vi "Stiffness Limits DAO.vi"(0 "Actions":T5, 3 "Config Ref Number":T4, 7 "ID":T3, 9 "Stiffness Limit In":T1, 11 "error in (no error)":errorcluster) -> (8 "Stiffness Limit Out":T1, 14 "Config Ref Number out":T4, 15 "error out":errorcluster)   [LabVIEW 2013]
uses:
  Metadata/Persistant DAO Actions.ctl
  <vilib>/Utility/config.llb/Config Data RefNum.ctl
  Metadata/LBCB Number.ctl
  Metadata/Cartesian Matrix.ctl
  Metadata/Cartesian Point.ctl
  <vilib>/Utility/config.llb/NI_LVConfig.lvlib
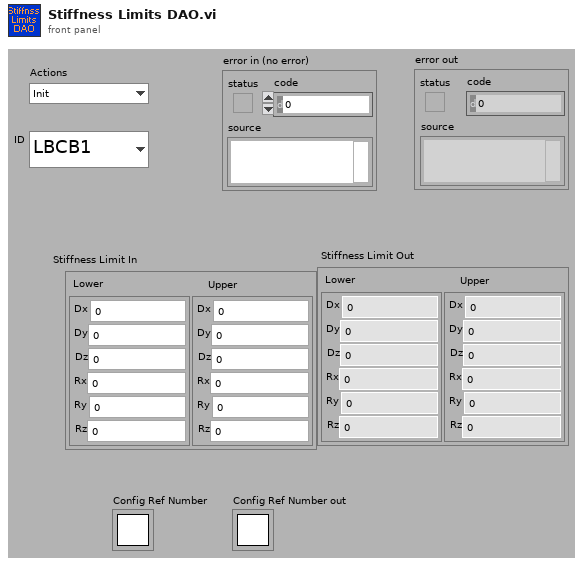
[diagram p1: front panel]
types:
  T1 = typedef "Cartesian Matrix.ctl" = cluster{"Lower":T2, "Upper":T2}
  T2 = typedef "Cartesian Point.ctl" = cluster{"Dx":dbl, "Dy":dbl, "Dz":dbl, "Rx":dbl, "Ry":dbl, "Rz":dbl}
  T3 = typedef "LBCB Number.ctl" = enum16{"LBCB1", "LBCB2"}
  T4 = typedef "NI_LVConfig.lvlib/Config Data RefNum.ctl" = refnum<k1>
  T5 = typedef "Persistant DAO Actions.ctl" = enum16{"Init", "Get", "Set", "Load", "Save"}
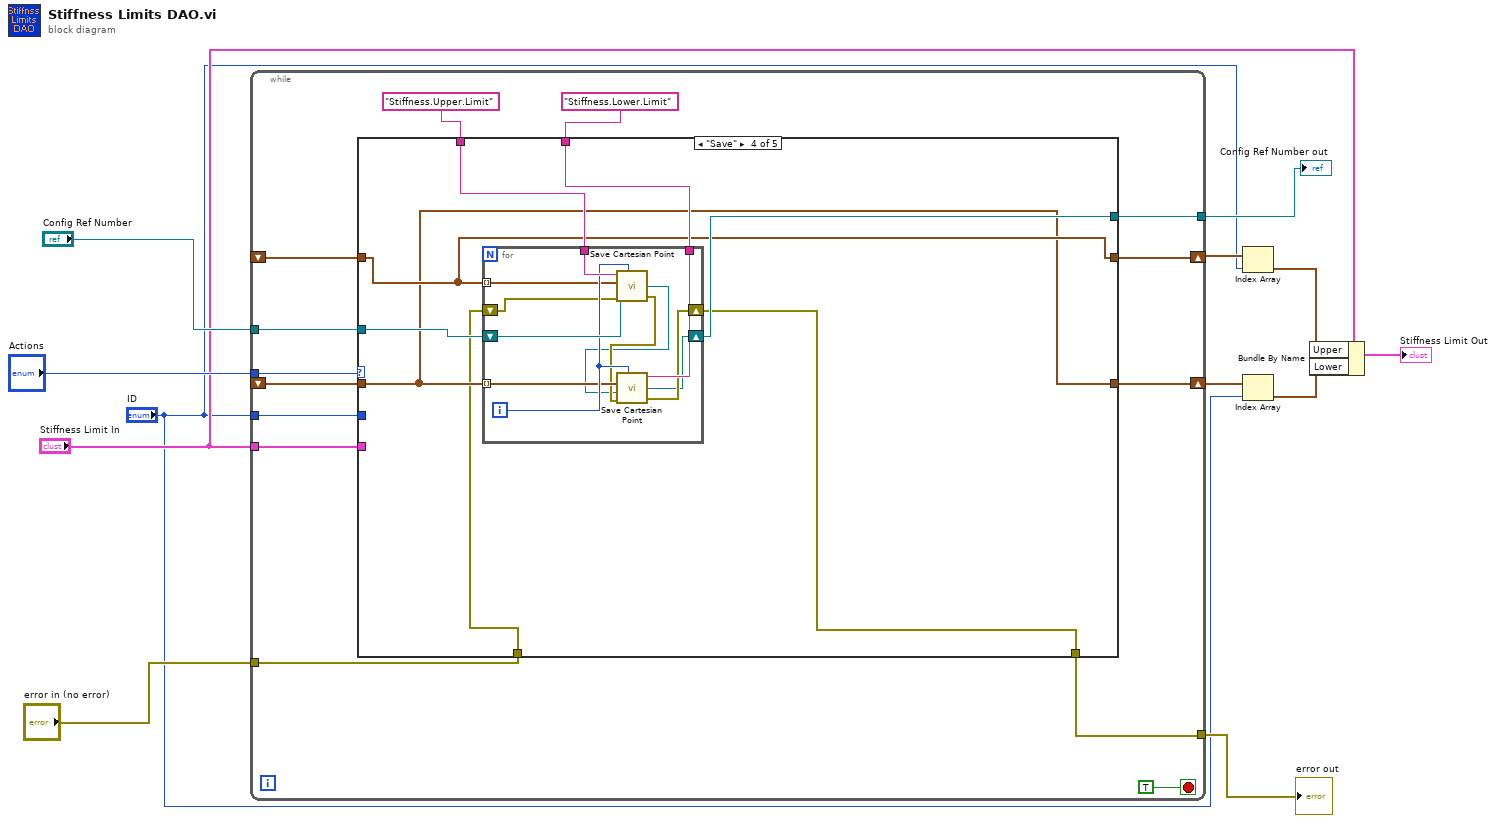
[diagram p0: block diagram]
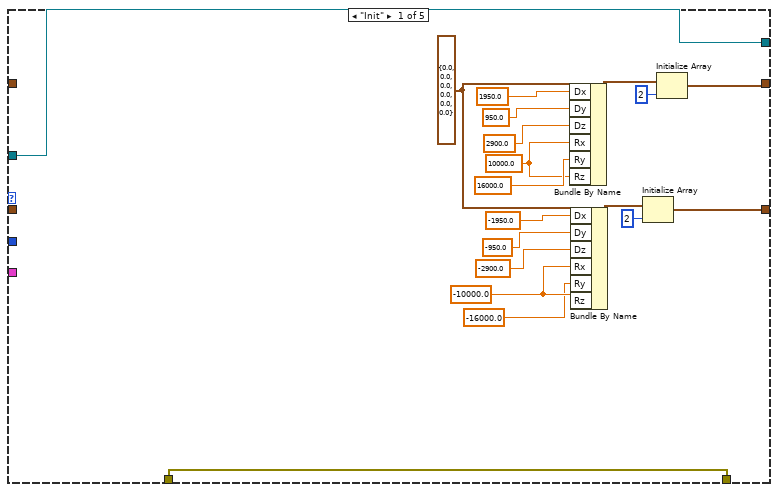
[diagram p2: hidden frame]
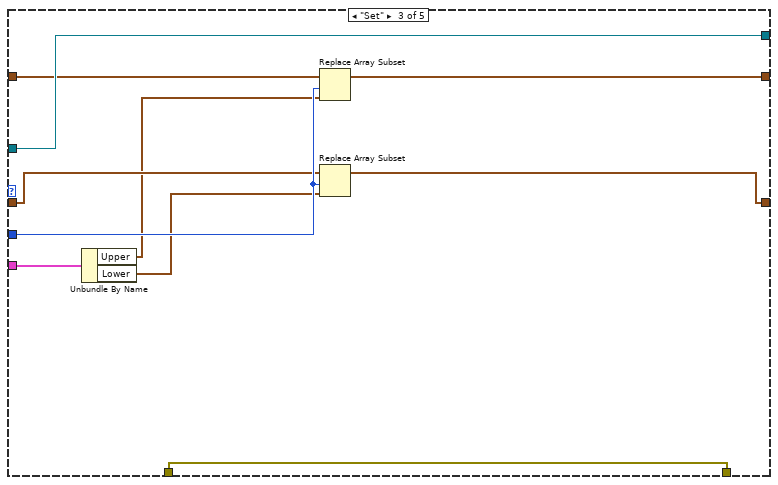
[diagram p4: hidden frame]
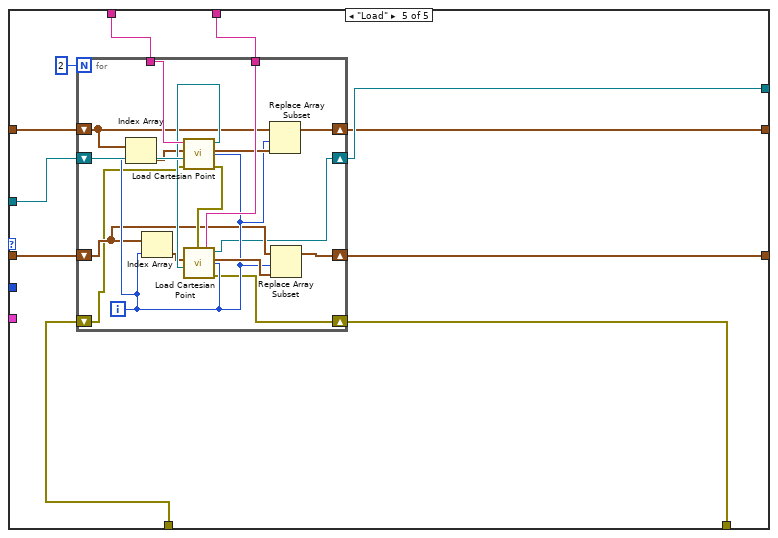
[diagram p5: hidden frame]
diagram:
  n1 = while {
    tunnel: "Actions" -> [w25]
    tunnel: "Config Ref Number" -> [w24]
    tunnel: "ID" -> [w21]
    tunnel: "error in (no error)" -> [w14]
    tunnel: [w20] -> w9
    tunnel: [w19] -> w8
    shift-right: [w17] -> w6
    shift-left: _ -> [w15]
    shift-right: [w18] -> w7
    shift-left: _ -> [w16]
    tunnel: "Stiffness Limit In" -> [w13]
    stop <- TRUE stop-if-true
    n2 = case shown="\"Save\"" w25 {
      tunnel: "Stiffness.Upper.Limit" ("section") -> [_ _ _ w66 w88]
      tunnel: w24 -> [w45 w49 w59 w67 w89]
      tunnel: "Stiffness.Lower.Limit" ("section") -> [_ _ _ w65 w87]
      tunnel: w21 -> [_ _ w58 _ _]
      tunnel: [w45 w49 w59 w64 w86] -> w20
      tunnel: [w40 w46 w50 w60 w79] -> w19
      tunnel: [w43 w48 w57 w63 w85] -> w18
      tunnel: [w41 w47 w56 w62 w84] -> w17
      tunnel: w16 -> [_ w48 w54 w63 w83]
      tunnel: w15 -> [_ w47 w55 w62 w82]
      tunnel: w14 -> [w40 w46 w50 w61 w80]
      tunnel: w13 -> [_ _ w53 _ _]
      frame "Init" {
        w38 = T2 {"Dx"=0.0, "Dy"=0.0, "Dz"=0.0, "Rx"=0.0, "Ry"=0.0, "Rz"=0.0} ("Upper")
        w28 = -10000.0 ("Rx")
        w32 = 10000.0 ("Rx")
        n3 = Bundle By Name(cluster=w38, "Dx"=1950.0 ("X"), "Dy"=950.0 ("Y"), "Dz"=2900.0 ("Z"), "Rx"=w32, "Ry"=16000.0, "Rz"=w32) -> (w39:T2)
        n4 = Bundle By Name(cluster=w38, "Dx"=-1950.0 ("X"), "Dy"=-950.0 ("Y"), "Dz"=-2900.0 ("Z"), "Rx"=w28, "Ry"=-16000.0, "Rz"=w28) -> (w37:T2)
        n5 = Initialize Array(w37, 2 ("dimension size")) -> (w41:T2[])
        n6 = Initialize Array(w39, 2 ("dimension size")) -> (w43:T2[])
      }
      frame "Get" {
      }
      frame "Set" {
        n7 = Unbundle By Name(w53) -> ("Upper"=w52:T2, "Lower"=w51:T2)
        n8 = Replace Array Subset(array=w54, new element=w52, index=w58) -> (w57:T2[])
        n9 = Replace Array Subset(array=w55, new element=w51, index=w58) -> (w56:T2[])
      }
      frame "Save" {
        n10 = for {
          tunnel: w66 -> [w77]
          tunnel: w65 -> [w76]
          shift-right: [w68] -> w64
          shift-left: w67 -> [w78]
          shift-right: [w70] -> w60
          shift-left: w61 -> [w72]
          tunnel: w63 -> [w74] mode=indexing
          tunnel: w62 -> [w73] mode=indexing
          i -> [w75]
          n11 = call "Save Cartesian Point.vi"("section"=w77, "Input Cluster"=w74, "refnum"=w78, "error in (no error)"=w72, "LBCB Number"=w75) -> ("refnum out"=w69:T4, "error out"=w71:errorcluster)  [unwired: 1 out]
          n12 = call "Save Cartesian Point.vi"("section"=w76, "Input Cluster"=w73, "refnum"=w69, "error in (no error)"=w71, "LBCB Number"=w75) -> ("refnum out"=w68:T4, "error out"=w70:errorcluster)  [unwired: 1 out]
        }
      }
      frame "Load" {
        n13 = for {
          N: 2 -> [_]
          tunnel: w88 -> [w105]
          tunnel: w87 -> [w103]
          shift-right: [w92] -> w86
          shift-left: w89 -> [w106]
          shift-right: [w98] -> w85
          shift-left: w83 -> [w94]
          shift-right: [w97] -> w84
          shift-left: w82 -> [w93]
          shift-right: [w90] -> w79
          shift-left: w80 -> [w91]
          i -> [w99]
          n14 = Index Array(array=w94, index=w99) -> (element=w96:T2)
          n15 = Index Array(array=w93, index=w99) -> (element=w95:T2)
          n16 = call "Load Cartesian Point.vi"("LBCB Number"=w99, "error in (no error)"=w91, "refnum"=w106, "Input Cluster"=w96, "section"=w105) -> ("error out"=w104:errorcluster, "output cluster"=w101:T2, "refnum out"=w102:T4)  [unwired: 1 out]
          n17 = call "Load Cartesian Point.vi"("LBCB Number"=w99, "error in (no error)"=w104, "refnum"=w102, "Input Cluster"=w95, "section"=w103) -> ("error out"=w90:errorcluster, "output cluster"=w100:T2, "refnum out"=w92:T4)  [unwired: 1 out]
          n18 = Replace Array Subset(array=w94, new element=w101, index=w99) -> (w98:T2[])
          n19 = Replace Array Subset(array=w93, new element=w100, index=w99) -> (w97:T2[])
        }
      }
    }
  }
  "error out" <- w8
  "Config Ref Number out" <- w9
  n20 = Index Array(array=w7, index="ID") -> (element=w4:T2)
  n21 = Index Array(array=w6, index="ID") -> (element=w3:T2)
  n22 = Bundle By Name(cluster="Stiffness Limit In", "Upper"=w4, "Lower"=w3) -> (→"Stiffness Limit Out":T1)
